vi "Callback - Shutdown.vi"(8 "error in (no error)":errorcluster, 11 "StokePlotHandle in":refnum<class "BjusticePlotHandle.lvclass">) -> (0 "error out":errorcluster, 3 "StokePlotHandle out":refnum<class "BjusticePlotHandle.lvclass">)   [LabVIEW 2021, in "BjusticePlotHandle.lvclass"]
uses:
  BjusticePlotHandle.lvclass
  BjusticePlotHandle.lvclass/BjusticePlotHandle.ctl
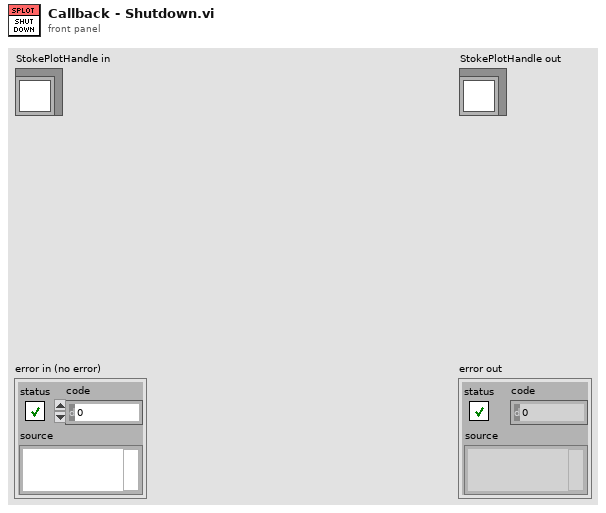
[diagram p1: front panel]
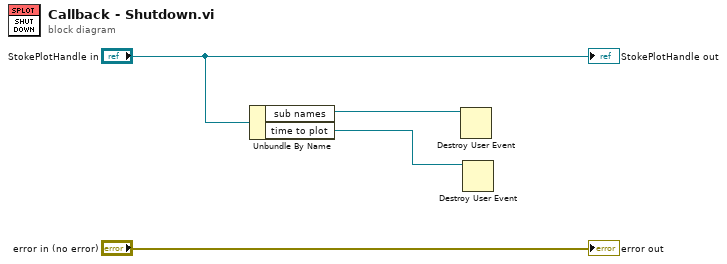
[diagram p0: block diagram]
diagram:
  n1 = Unbundle By Name("StokePlotHandle in") -> ("sub names"=w2:refnum<user-event>, "time to plot"=w1:refnum<user-event>)
  n2 = Destroy User Event(user event=w2) -> ()  [unwired: 1 in, 1 out]
  n3 = Destroy User Event(user event=w1) -> ()  [unwired: 1 in, 1 out]
  "error out" <- "error in (no error)"
  "StokePlotHandle out" <- "StokePlotHandle in"
